vi "Attach GUI Controls.vi"(8 "error in (no error)":errorcluster, 10 "GUI Control.lvclass":refnum<class "GUI Control.lvclass">, 11 "Panel GUI Manager in":refnum<class "Panel GUI Manager.lvclass">) -> (0 "error out":errorcluster, 3 "Panel GUI Manager out":refnum<class "Panel GUI Manager.lvclass">)   [LabVIEW 2015, in "Panel GUI Manager.lvclass"]
uses:
  Panel GUI Manager.lvclass
  GUI/GUI Controls/GUI Control/GUI Control.lvclass
  Panel GUI Manager.lvclass/Panel GUI Manager.ctl
  GUI/GUI Controls/GUI Control/GUI Control.lvclass/GUI Control.ctl
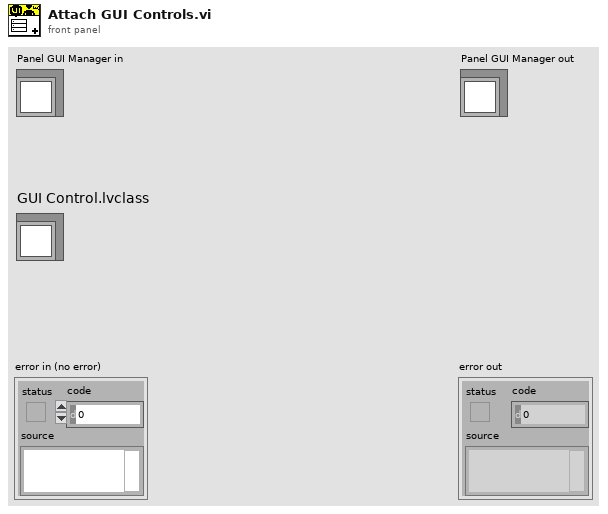
[diagram p1: front panel]
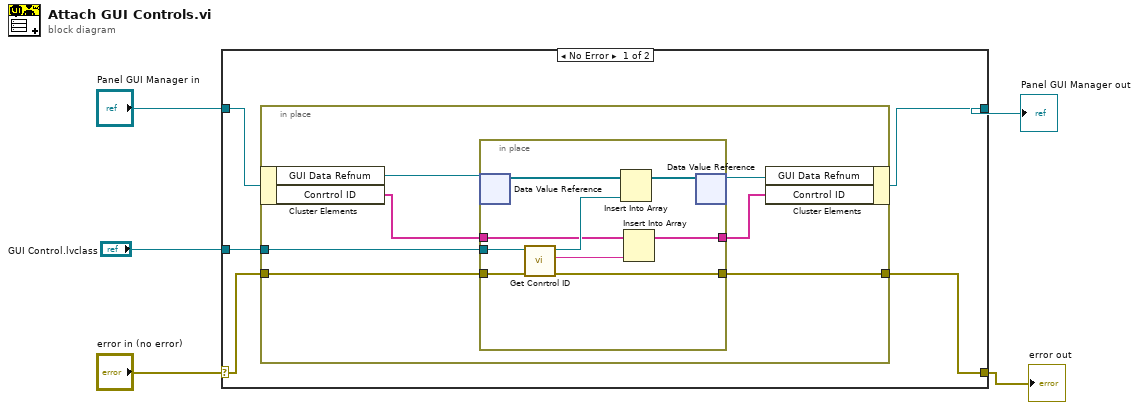
[diagram p0: block diagram]
diagram:
  n1 = case shown="No Error" "error in (no error)" {
    selector: "error in (no error)" -> [w9 w28]
    tunnel: [w6 w28] -> w4
    tunnel: [w7 w27] -> w2
    tunnel: "Panel GUI Manager in" -> [w8 w27]
    tunnel: "GUI Control.lvclass" -> [w10 _]
    frame No Error {
      n2 = in-place {
        in-place-border: w10 -> [w17]
        in-place-border: w9 -> [w16]
        in-place-border: [w13] -> w6
        n3 = in-place-cluster #1(w8) -> ("GUI Data Refnum"=w12:refnum<data-value>, "Conrtrol ID"=w11:string[])
        n4 = in-place {
          in-place-border: w17 -> [w25]
          in-place-border: w16 -> [w24]
          in-place-border: [w20] -> w14
          in-place-border: [w19] -> w13
          in-place-border: w11 -> [w18]
          n5 = in-place-dvr #2(w12) -> (w26:refnum<class "GUI Control.lvclass">[])  [unwired: 1 out]
          n6 = call "Get Conrtrol ID.vi"("error in (no error)"=w24, "GUI Control in"=w25) -> ("error out"=w19:errorcluster, "Control ID"=w21:string, "GUI Control out"=w23:refnum<class "GUI Control.lvclass">)  [unwired: 7 in]
          n7 = Insert Into Array(array=w26, new element=w23) -> (w22:refnum<class "GUI Control.lvclass">[])  [unwired: 1 in]
          n8 = Insert Into Array(array=w18, new element=w21) -> (w20:string[])  [unwired: 1 in]
          n9 = in-place-dvr #2(w22) -> (w15:refnum<data-value>)  [unwired: 1 out]
        }
        n10 = in-place-cluster #1("GUI Data Refnum"=w15, "Conrtrol ID"=w14) -> (w7:refnum<class "Panel GUI Manager.lvclass">)
      }
    }
    frame Error {
    }
  }
  "error out" <- w4
  "Panel GUI Manager out" <- w2
